vi "Lockin_AIWFM_time.vi"(8 "error in (no error)":errorcluster, 11 "Transport":refnum<class "Transport.lvclass">) -> (0 "error out":errorcluster, 3 "Transport out":refnum<class "Transport.lvclass">)   [LabVIEW 2019, in "Transport.lvclass"]
uses:
  Transport.lvclass
  <userlib>/LevyLab/Instrument Framework/Instrument Types/Cryostat/Instrument.Cryostat.lvclass
  Control Experiment/Control Experiment.lvclass
  Control Experiment/Typedefs/Instrument Classes--cluster.ctl
  <userlib>/LevyLab/Instrument Framework/Instrument Types/VSource/Instrument.VSource.lvclass
  <userlib>/LevyLab/Instrument Framework/Instrument Types/VNA/Instrument.VNA.lvclass
  <userlib>/LevyLab/Instrument Framework/Instrument Types/Strain/Instrument.Strain.lvclass
  <userlib>/LevyLab/Instrument Framework/Instrument Types/CBridge/Instrument.CBridge.lvclass
  <vilib>/Waveform/WDTOps.llb/WDT Append Waveforms DBL.vi
  <vilib>/PRIrvin/XY Utilities/xy_utilities.lvlib
  <vilib>/PRIrvin/XY Utilities/subVIs/Waveform to XY (single).vi
  <vilib>/PRIrvin/XY Utilities/subVIs/Get X and Y (single).vi
  <userlib>/LevyLab/Instrument Framework/Instrument Types/Delay Line/Instrument.DelayLine.lvclass
  <userlib>/LevyLab/Instrument Framework/Instrument Types/Lockin/Instrument.LockinAPI.lvclass
  <userlib>/LevyLab/Instrument Framework/Instrument Types/Amplifier/Instrument.Amplifier.lvclass
panel:
  in  "Stop":bool
  in  "Tab Control":enum32{"Control", "Waveform", "Other"}(tab)
  in  "wait (ms)":u32=1000
  in  "Experiment Description":string="cool down\n\n"
  in  "Experiment Folder":string="cooldown"
  out "AI":cluster{dbl[], dbl[]}[](graph)
  # "*** These controls are only read if this VI is the top level. If is is called from Sweep Control then the folder and comments come from Sweep Control.vi ***"
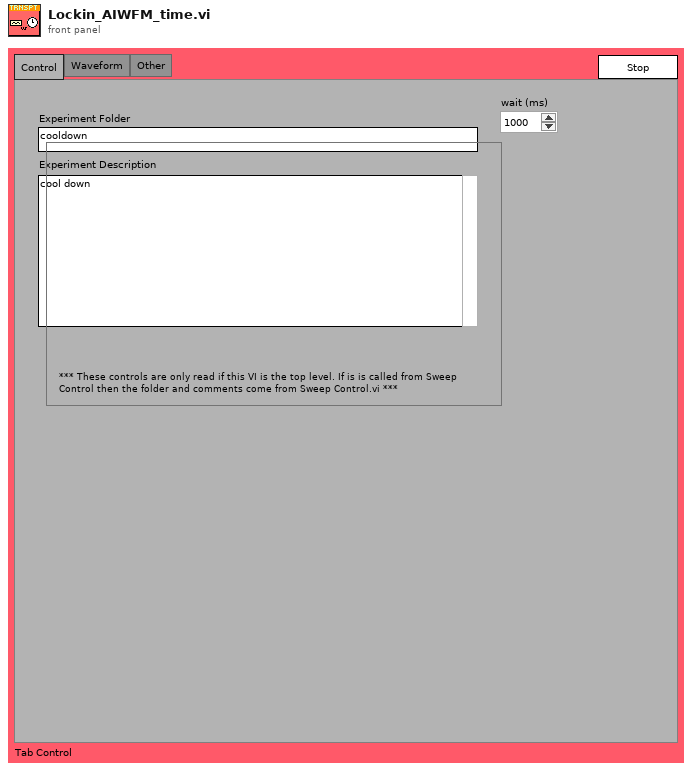
[diagram p1: front panel]
types:
  T1 = enum32{"Invalid", "Standard", "Closed", "Hidden", "Minimized", "Maximized"}
  T2 = enum32{"invalid app kind", "Development System", "Run Time System", "Student Edition", "Embedded LabVIEW", "Evaluation", "Custom"}
  T3 = typedef "Control Experiment.lvclass/Instrument Classes--cluster.ctl" = cluster{"DAQ":refnum<class "Instrument.LockinAPI.lvclass">, "Amplifier":refnum<class "Instrument.Amplifier.lvclass">, "Temperature":refnum<class "Instrument.Cryostat.lvclass">, "Magnet":refnum<class "Instrument.Cryostat.lvclass">, "Rotator":refnum<class "Instrument.Cryostat.lvclass">, "Level":refnum<class "Instrument.Cryostat.lvclass">, "Capacitance":refnum<class "Instrument.CBridge.lvclass">, "Delay Line":refnum<class "Instrument.DelayLine.lvclass">, "Strain Cell":refnum<class "Instrument.Strain.lvclass">, "VNA":refnum<class "Instrument.VNA.lvclass">, "Source":refnum<class "Instrument.VSource.lvclass">}
  T4 = cluster{"Core":cluster{"Current VI Reference":refnum<vi>, "Close Panel on Exit?":bool}, "Transport":refnum<class "Transport.lvclass">, "C.E.":refnum<class "Control Experiment.lvclass">, "Notifier":refnum<notifier>, "Instruments":T3, "path":path, "time":dbl, "temperature":dbl, "magnet field":dbl, "AI XY (new)":cluster{dbl[], dbl[]}[], "AI XY (all)":cluster{dbl[], dbl[]}[], "AI Waveform (s)":waveform(dbl)[], "t0":timestamp, "Execution:State":enum32{"Bad", "Idle", "Run top level", "Running"}}
  T5 = enum32{"Bad", "Idle", "Run top level", "Running"}
  T6 = cluster{"Current VI Reference":refnum<vi>, "Close Panel on Exit?":bool}
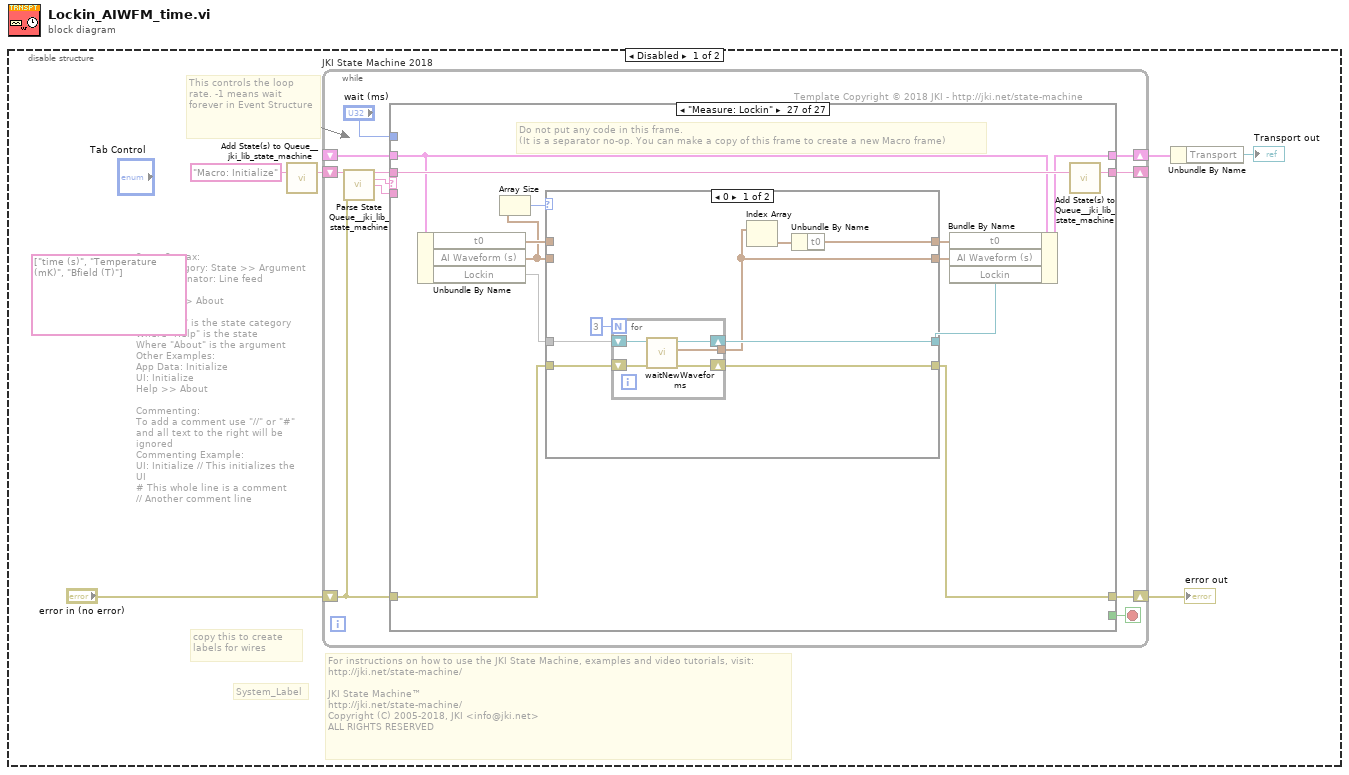
[diagram p0: block diagram]
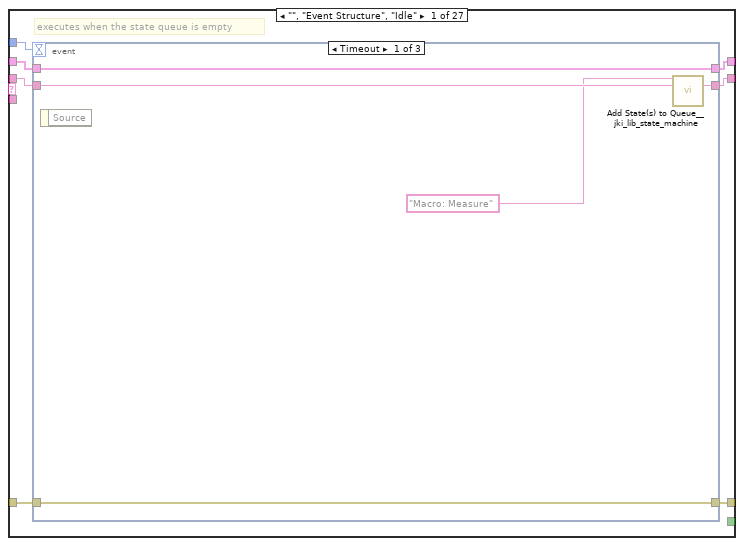
[diagram p2: hidden frame]
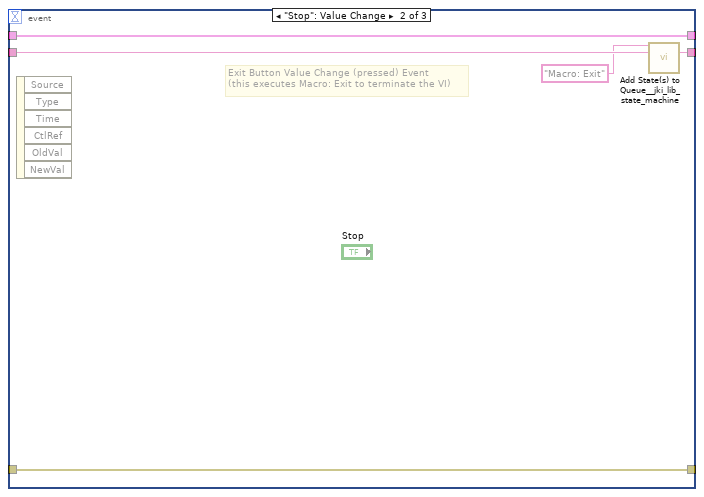
[diagram p3: hidden frame]
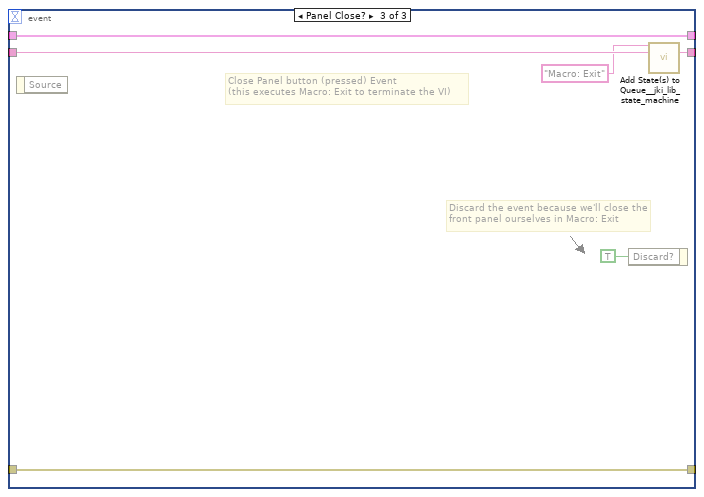
[diagram p4: hidden frame]
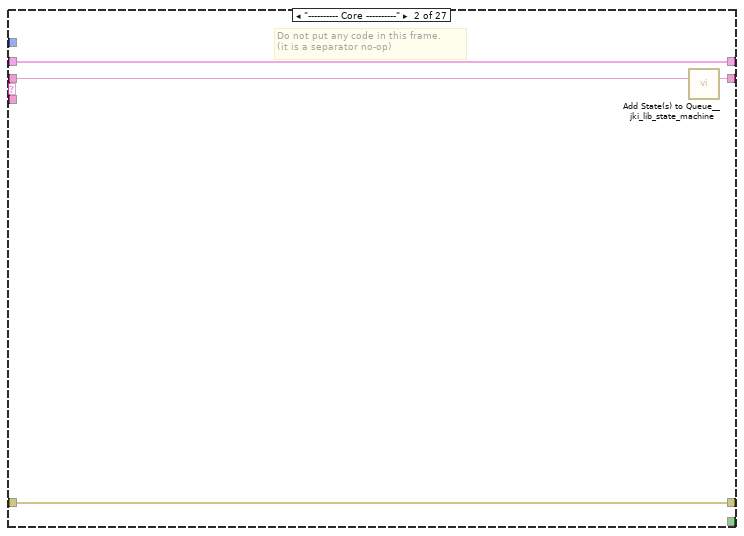
[diagram p5: hidden frame]
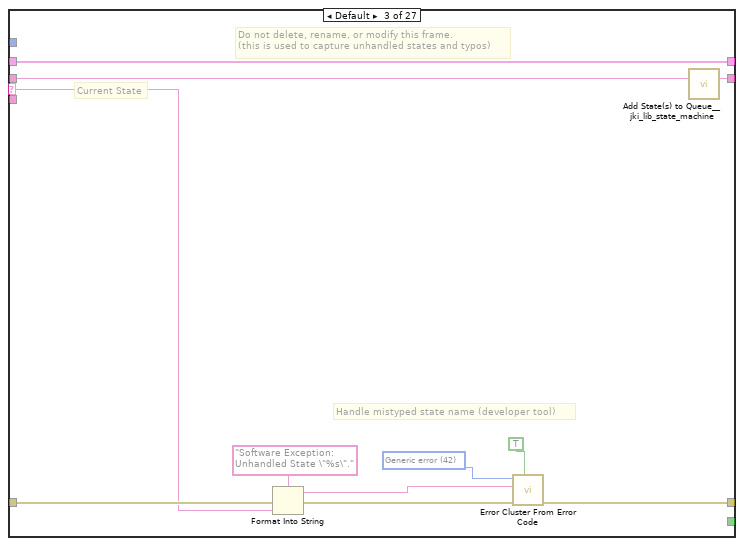
[diagram p6: hidden frame]
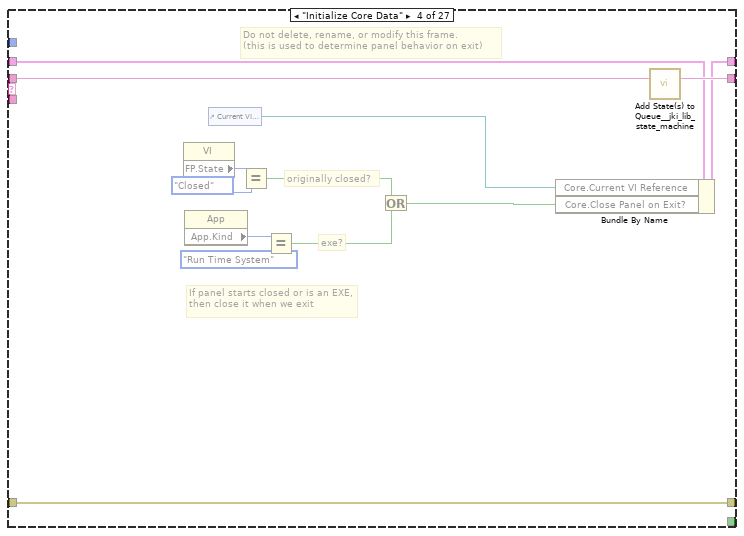
[diagram p7: hidden frame]
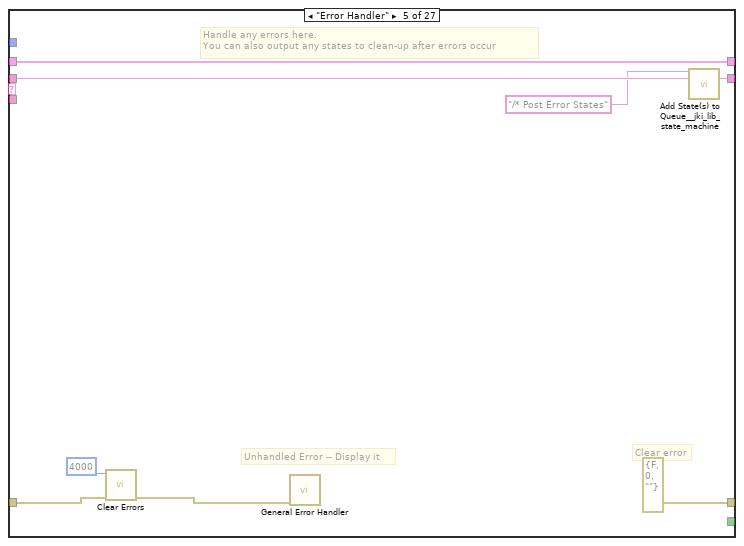
[diagram p8: hidden frame]
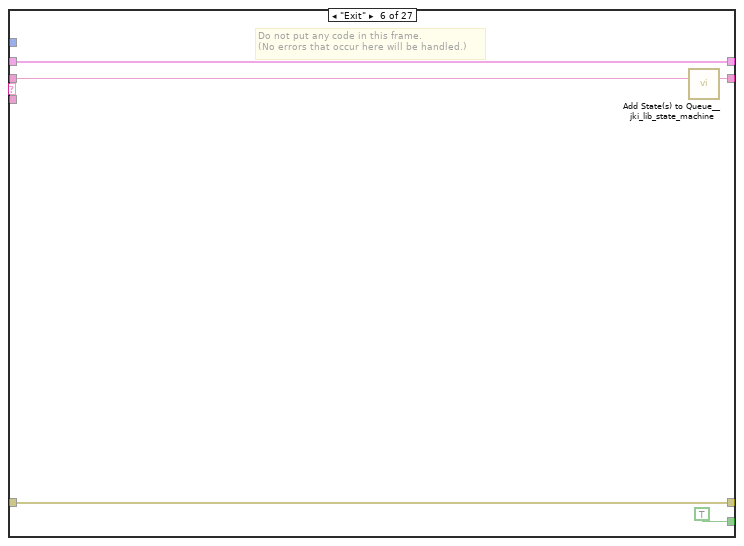
[diagram p9: hidden frame]
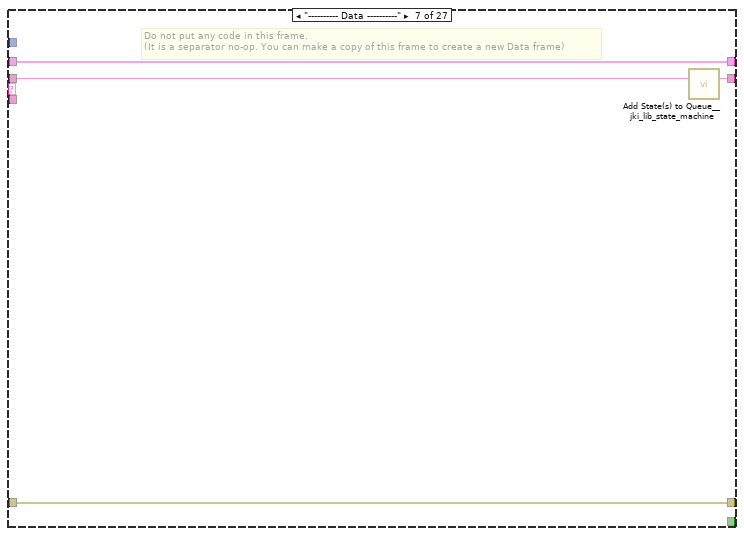
[diagram p10: hidden frame]
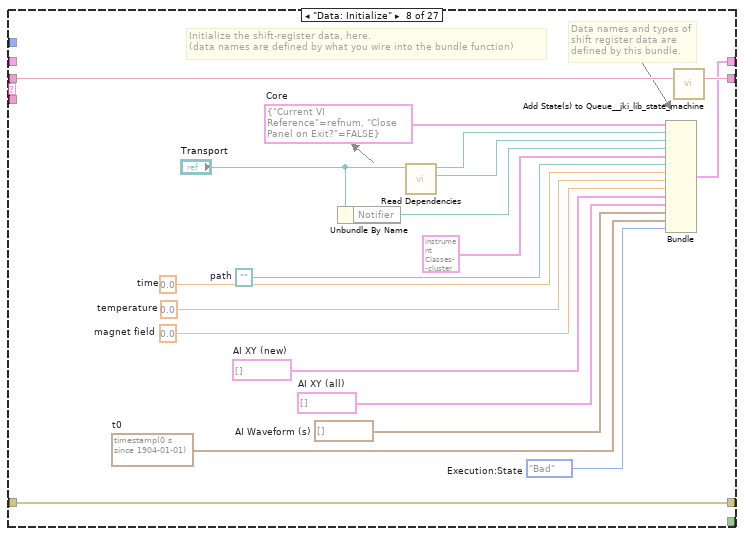
[diagram p11: hidden frame]
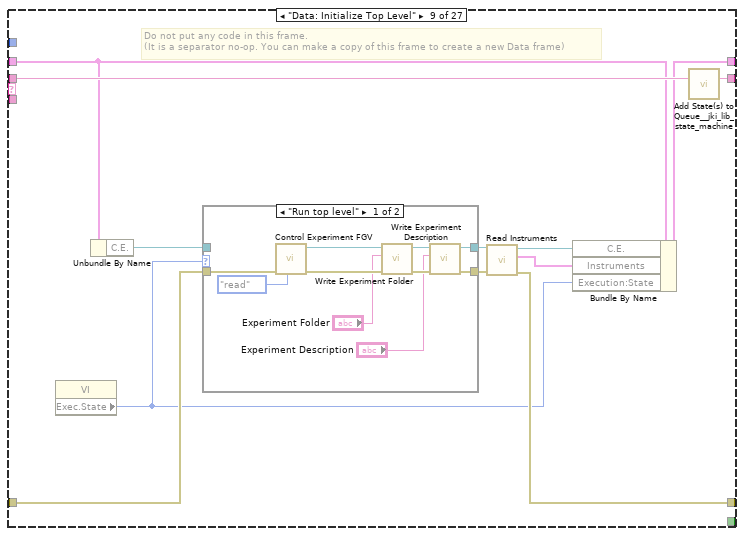
[diagram p12: hidden frame]
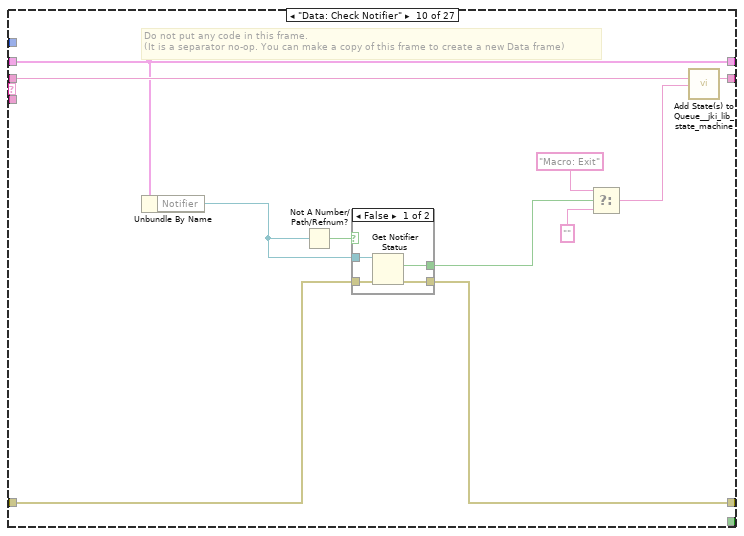
[diagram p14: hidden frame]
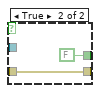
[diagram p15: hidden frame]
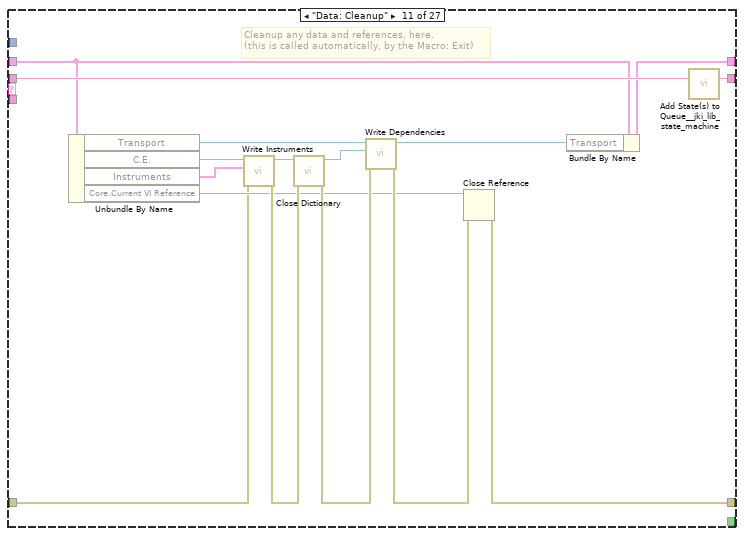
[diagram p16: hidden frame]
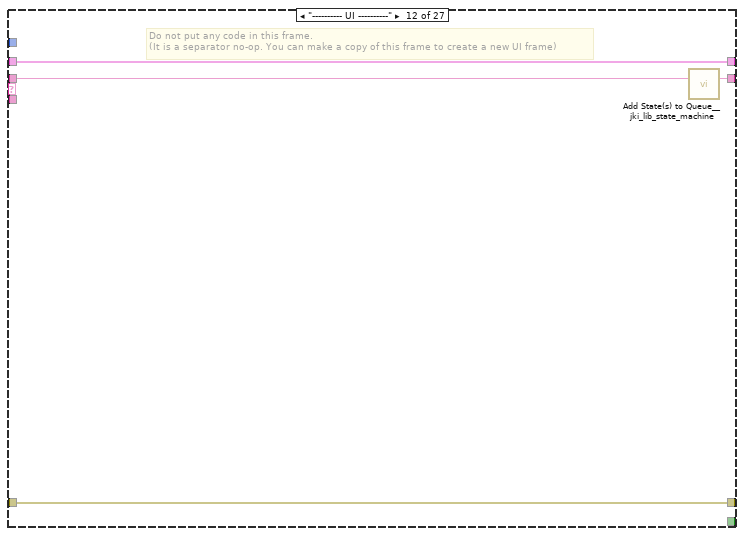
[diagram p17: hidden frame]
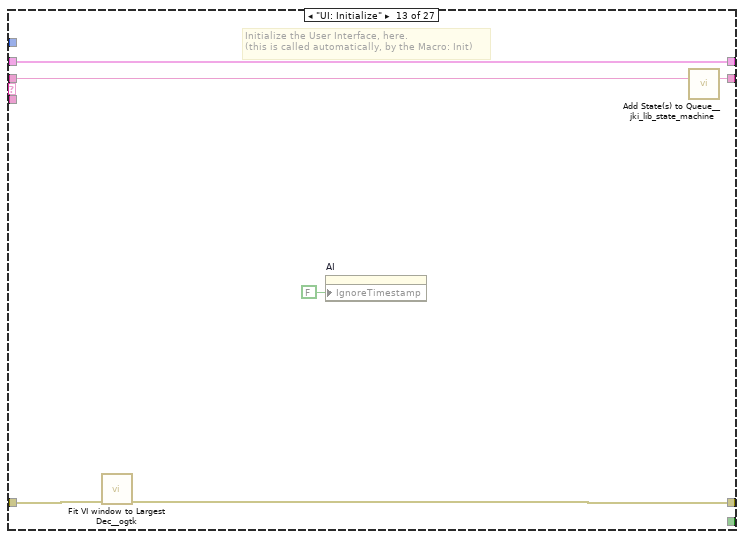
[diagram p18: hidden frame]
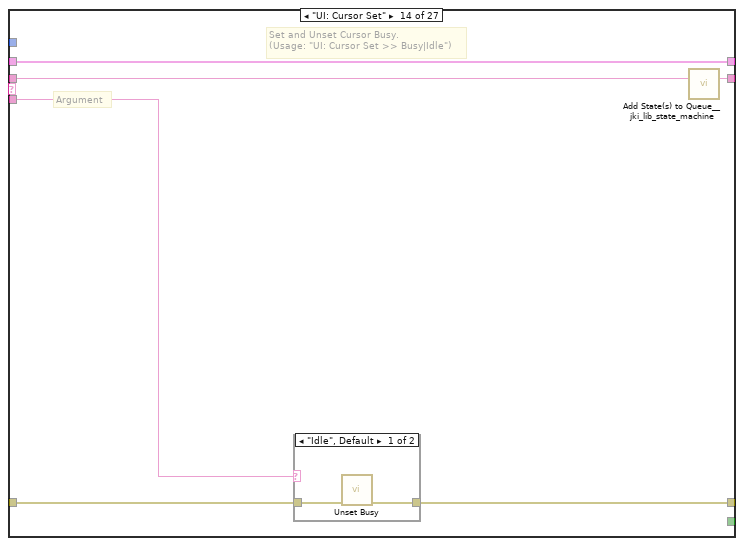
[diagram p19: hidden frame]
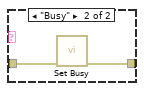
[diagram p20: hidden frame]
diagram:
  n1 = disable-structure shown="Disabled" {
    frame Disabled {
      (unwired) string[] ["time (s)", "Temperature (mK)", "Bfield (T)"] ("wavenames (.Vx, etc)")
      # "For instructions on how to use the JKI State Machine, examples and video tutorials, visit:\nhttp://jki.net/state-machine/\n\nJKI State Machine™\nhttp://jki.net/state-machine/\nCopyright (C) 2005-2018, JKI <info@jki.net>\nALL RIGHTS RESERVED"
      # "State Syntax:\nStateCategory: State >> Argument\nLine Terminator: Line feed\nExample:\nUI: Help >> About\n\nWhere \"UI\" is the state category\nWhere \"Help\" is the state\nWhere \"About\" is the argument\nOther Examples:\nApp Data: Initialize\nUI: Initialize\nHelp >> About\n\nCommenting:\nTo add a comment use \"//\" or \"#\" and all text to the right will be ignored\nCommenting Example:\nUI: Initialize // This initializes the UI\n# This whole line is a comment\n// Another comment line"
      # "copy this to create labels for wires"
      # "This controls the loop rate. -1 means wait forever in Event Structure"
      # "System_Label"
      n2 = call <vilib>:"Add State(s) to Queue__jki_lib_state_machine.vi"("State(s) in (\"\")"="Macro: Initialize") -> ("States Out"=w6:string)  [unwired: 14 in]
      n3 = while "JKI State Machine 2018" {
        shift-right: [w10] -> w2
        shift-left: _ -> [w9]
        shift-right: [w13] -> w3
        shift-left: "error in (no error)" -> [w8]
        shift-right: [w12] -> _
        shift-left: w6 -> [w14]
        stop <- w11 stop-if-true
        # "Template Copyright © 2018 JKI - http://jki.net/state-machine"
        n4 = call <vilib>:"Parse State Queue__jki_lib_state_machine.vi"("State Queue"=w14, "Error In (no error)"=w8) -> ("Remaining States"=w16:string, "Current State"=w17:string, "Arguments"=w15:string)  [unwired: 11 in]
        n5 = case shown="\"Measure: Lockin\"" w17 {
          selector: w17 -> [_ _ w45 _ _ _ _ _ _ _ _ _ _ _ _ _ _ _ _ _ _ _ _ _ _ _ _]
          tunnel: w16 -> [w24 w44 w49 w68 w76 w81 w85 w104 w116 w139 w161 w165 w171 w177 w188 w258 w262 w267 w275 w285 w289 w303 w327 w338 w351 w364 w377]
          tunnel: w15 -> [_ _ _ _ _ _ _ _ _ _ _ _ _ w172 w182 _ _ _ _ _ _ _ _ _ _ _ _]
          tunnel: w9 -> [w22 w41 w47 w61 w73 w79 w82 _ w112 w136 w146 w162 w169 w175 w184 w256 w259 w264 w272 w282 w286 w292 w324 w334 w347 w362 w374]
          tunnel: [w21 w42 w51 w65 errorcluster {"status"=FALSE, "code"=0, "source"=""} ("error out") w78 w83 w101 w106 w135 w148 w163 w167 w173 w185 w255 w260 w265 w273 w283 w287 w301 w325 w328 w340 w357 w368] -> w13
          tunnel: w8 -> [w20 w42 w50 w65 w70 w78 w83 w101 w111 w134 w149 w163 w168 w174 w186 w255 w260 w265 w273 w283 w287 w296 w325 w331 w348 w356 w369]
          tunnel: [w23 w43 w48 w67 w75 w80 w84 w103 w115 w138 w160 w164 w170 w176 w187 w257 w261 w266 w274 w284 w288 w302 w326 w337 w350 w363 w376] -> w12
          tunnel: [_ _ _ _ _ TRUE _ _ _ _ _ _ _ _ _ _ _ _ _ _ _ _ _ _ _ _ _] -> w11
          tunnel: [w19 w41 w47 w66 w73 w79 w82 w102 w113 w136 w147 w162 w169 w175 w184 w256 w259 w264 w272 w282 w286 w291 w324 w335 w346 w361 w375] -> w10
          tunnel: "wait (ms)" -> [w18 _ _ _ _ _ _ _ _ _ _ _ _ _ _ _ _ _ _ _ _ _ _ _ _ _ _]
          frame "", "Event Structure", "Idle" {
            # "executes when the state queue is empty"
            n6 = event shown="[0] Timeout" {
              selector: _ -> [_ _ _]
              dyn-events: _ -> [_ _ _]
              timeout: w18 -> [_ _ _]
              tunnel: w24 -> [w29 w34 w40]
              tunnel: [w28 w33 w39] -> w23
              tunnel: w22 -> [w26 w31 w37]
              tunnel: [w27 w32 w38] -> w21
              tunnel: w20 -> [w27 w32 w38]
              tunnel: [w26 w31 w37] -> w19
              event Timeout {
                n7 = event-data() -> ()  [unwired: 1 in, 1 out]
                n8 = call <vilib>:"Add State(s) to Queue__jki_lib_state_machine.vi"("State(s) in Front (\"\")"="Macro: Measure" ("State(s) in Front (\"\")"), "State(s) in (\"\")"=w29) -> ("States Out"=w28:string)  [unwired: 13 in]
              }
              event "Stop": Value Change {
                # "Exit Button Value Change (pressed) Event\n(this executes Macro: Exit to terminate the VI)"
                n9 = event-data() -> ()  [unwired: 1 in, 6 out]
                n10 = call <vilib>:"Add State(s) to Queue__jki_lib_state_machine.vi"("State(s) in Front (\"\")"="Macro: Exit", "State(s) in (\"\")"=w34) -> ("States Out"=w33:string)  [unwired: 13 in]
              }
              event Panel Close? {
                # "Discard the event because we'll close the front panel ourselves in Macro: Exit"
                # "Close Panel button (pressed) Event\n(this executes Macro: Exit to terminate the VI)"
                n11 = event-data() -> ()  [unwired: 1 in, 1 out]
                n12 = event-data("Discard?"=TRUE) -> ()  [unwired: 1 in, 1 out]
                n13 = call <vilib>:"Add State(s) to Queue__jki_lib_state_machine.vi"("State(s) in Front (\"\")"="Macro: Exit", "State(s) in (\"\")"=w40) -> ("States Out"=w39:string)  [unwired: 13 in]
              }
            }
          }
          frame "---------- Core ----------" {
            # "Do not put any code in this frame.\n(it is a separator no-op)"
            n14 = call <vilib>:"Add State(s) to Queue__jki_lib_state_machine.vi"("State(s) in (\"\")"=w44) -> ("States Out"=w43:string)  [unwired: 14 in]
          }
          frame Default {
            w54 = 42 items=["No error", "Argument error", "Memory is full", "Out of zone", "End of file", "File already open", "Generic file I/O error", "File not found", "File permission error", "Disk is full", "Duplicate path", "Too many files open", "System feature not enabled", "Resource file not found", "Cannot add resource", "Resource not found", "Image not found", "Image memory error", "Pen does not exist", "Config type invalid", "Config token not found", "Config parse error", "Config memory error", "Bad external code format", "Bad external code offset", "External code not present", "Null window", "Destroy window error", "Null menu", "Print aborted", "Bad print record", "Print driver error", "Windows error during printing", "Memory error during printing", "Print dialog error", "Generic print error", "Invalid device refnum", "Device not found", "Device parameter error", "Device unit error", "Cannot open device", "Device call aborted", "Generic error", "Cancelled by user", "Object ID too low", "Object ID too high", "Object not in heap", "Unknown heap", "Unknown object (invalid DefProc)", "Unknown object (DefProc not in table)", "Message out of range", "Invalid (null) method", "Unknown message", "Manager call not supported", "Bad address", "Network operation in progress", "Network operation timed out", "Connection is busy", "Network attribute not supported", "Network error", "Address in use", "System out of memory", "Connection aborted", "Connection refused", "Not connected", "Already connected", "Connection closed", "Initialization error (interapplication manager)", "Bad occurrence", "Wait on unbound occurrence handler", "Occurrence queue overflow", "Datalog type conflict", "Unused", "Unrecognized type (interapplication manager)", "Memory corrupt", "Failed to make temporary DLL", "Old CIN version", "Drag socket not found", "Failed to load drop-object", "Failed to register OLE object", "Failed to release OLE object", "Format specifier type mismatch", "Unknown format specifier", "Too few format specifiers", "Too many format specifiers", "Scan failed", "Newer CIN version", "Error converting to variant", "Runtime menu error", "Password tampered", "Variant attribute not found", "Incompatible variant data type", "Event data is not available", "Event Store is not present", "Occurrence is not found", "Event Queue is not created", "Event info is not available", "Refnum passed is NULL", "Error retrieving Class GUID", "Error retrieving CoClass GUID", "Error retrieving TypeLib GUID.", "Bad built application magic bytes.", "Specific driver is different from the specific driver associated with the Logical Name.", "There is no session opened to the class driver.", "Max Error", "MAX - Error with config objects", "MAX - Error loading configuration", "MAX - Group not supported"]
            # "Current State"
            # "Do not delete, rename, or modify this frame.\n(this is used to capture unhandled states and typos)"
            # "Handle mistyped state name (developer tool)"
            n15 = Format Into String(format string="Software Exception: Unhandled State \"%s\"." ("message"), error in=w50, w45) -> (resulting string=w53:string, error out=w52:errorcluster)  [unwired: 1 in]
            n16 = call <vilib>:"Error Cluster From Error Code.vi"("show call chain? (False)"=TRUE, "error in (no error)"=w52, "error message (\"\")"=w53, "error code (0)"=w54) -> ("error out"=w51:errorcluster)  [unwired: 5 in]
            n17 = call <vilib>:"Add State(s) to Queue__jki_lib_state_machine.vi"("State(s) in (\"\")"=w49) -> ("States Out"=w48:string)  [unwired: 14 in]
          }
          frame "Initialize Core Data" {
            # "Do not delete, rename, or modify this frame.\n(this is used to determine panel behavior on exit)"
            # "originally closed?"
            # "exe?"
            # "If panel starts closed or is an EXE, then close it when we exit"
            n18 = property class="VI"() -> ("FP.State"=w58:T1)  [unwired: 2 in, 2 out]
            n19 = property class="App"() -> ("App.Kind"=w64:T2)  [unwired: 2 in, 2 out]
            n20 = control-ref of="Current VI Reference"() -> (w59:refnum<vi>)
            n21 = Equal?(x=w58, y=T1."Closed" ("Front Panel Window:State")) -> (x = y?=w56:bool)
            n22 = Equal?(x=w64, y=T2."Run Time System" ("Application:Kind")) -> (x = y?=w62:bool)
            n23 = Or(x=w56, y=w62) -> (x .or. y?=w60:bool)
            n24 = Bundle By Name(cluster=w61, "Core.Current VI Reference"=w59, "Core.Close Panel on Exit?"=w60) -> (w66:T4)
            n25 = call <vilib>:"Add State(s) to Queue__jki_lib_state_machine.vi"("State(s) in (\"\")"=w68) -> ("States Out"=w67:string)  [unwired: 14 in]
          }
          frame "Error Handler" {
            # "Unhandled Error -- Display it"
            # "Handle any errors here.\nYou can also output any states to clean-up after errors occur"
            # "Clear error"
            n26 = call <vilib>:"Clear Errors.vi"("error in (no error)"=w70, "specific error code to clear (0: all)"=4000) -> ("error out"=w69:errorcluster)  [unwired: 4 in, 1 out]
            n27 = call <vilib>:"General Error Handler.vi"("error in (no error)"=w69) -> ()  [unwired: 10 in, 5 out]
            n28 = call <vilib>:"Add State(s) to Queue__jki_lib_state_machine.vi"("State(s) in Front (\"\")"="/* Post Error States", "State(s) in (\"\")"=w76) -> ("States Out"=w75:string)  [unwired: 13 in]
          }
          frame "Exit" {
            # "Do not put any code in this frame.\n(No errors that occur here will be handled.)"
            n29 = call <vilib>:"Add State(s) to Queue__jki_lib_state_machine.vi"("State(s) in (\"\")"=w81) -> ("States Out"=w80:string)  [unwired: 14 in]
          }
          frame "---------- Data ----------" {
            # "Do not put any code in this frame.\n(It is a separator no-op. You can make a copy of this frame to create a new Data frame)"
            n30 = call <vilib>:"Add State(s) to Queue__jki_lib_state_machine.vi"("State(s) in (\"\")"=w85) -> ("States Out"=w84:string)  [unwired: 14 in]
          }
          frame "Data: Initialize" {
            w89 = T5."Bad"  # Execution:State
            w90 = timestamp(0 s since 1904-01-01)  # t0
            w91 = waveform(dbl)[] []  # AI Waveform (s)
            w96 = cluster{dbl[], dbl[]}[] []  # AI XY (new)
            w97 = cluster{dbl[], dbl[]}[] []  # AI XY (all)
            w94 = 0.0  # magnet field
            w93 = 0.0  # temperature
            w92 = 0.0  # time
            w99 = path ""  # path
            w100 = T6 {"Current VI Reference"=refnum, "Close Panel on Exit?"=FALSE}  # Core
            # "Data names and types of shift register data are defined by this bundle."
            # "Initialize the shift-register data, here.\n(data names are defined by what you wire into the bundle function)"
            n31 = Unbundle By Name("Transport") -> ("Notifier"=w98:refnum<notifier>)
            n32 = call "Read Dependencies.vi"("Transport"="Transport") -> ("C.E."=w86:refnum<class "Control Experiment.lvclass">, "Transport"=w87:refnum<class "Transport.lvclass">)  [unwired: 8 in, 1 out]
            n33 = Bundle("Core"=w100, "Transport"=w87, "C.E."=w86, "Notifier"=w98, "Instruments"=T3 {"DAQ"=refnum, "Amplifier"=refnum, "Temperature"=refnum, "Magnet"=refnum, "Rotator"=refnum, "Level"=refnum, "Capacitance"=refnum, "Delay Line"=refnum, "Strain Cell"=refnum, "VNA"=refnum, "Source"=refnum}, "path"=w99, "time"=w92, "temperature"=w93, "magnet field"=w94, "AI XY (new)"=w96, "AI XY (all)"=w97, "AI Waveform (s)"=w91, "t0"=w90, "Execution:State"=w89) -> (w102:T4)  [unwired: 1 in]
            n34 = call <vilib>:"Add State(s) to Queue__jki_lib_state_machine.vi"("State(s) in (\"\")"=w104) -> ("States Out"=w103:string)  [unwired: 14 in]
          }
          frame "Data: Initialize Top Level" {
            # "Do not put any code in this frame.\n(It is a separator no-op. You can make a copy of this frame to create a new Data frame)"
            n35 = property class="VI"() -> ("Exec.State"=w105:T5)  [unwired: 2 in, 2 out]
            n36 = Unbundle By Name(w112) -> ("C.E."=w114:refnum<class "Control Experiment.lvclass">)
            n37 = case shown="\"Run top level\"" w105 {
              tunnel: w111 -> [w126 w127]
              tunnel: [w121 w127] -> w110
              tunnel: [w120 w128] -> w109
              tunnel: w114 -> [_ w128]
              frame "Run top level" {
                n38 = call "Control Experiment FGV.vi"("Function"=enum16{"read", "write"}."read", "error in (no error)"=w126) -> ("error out"=w124:errorcluster, "Control Experiment.lvclass out"=w125:refnum<class "Control Experiment.lvclass">)  [unwired: 8 in]
                n39 = call "Write Experiment Folder.vi"("error in (no error)"=w124, "Experiment Folder"="Experiment Folder", "Control Experiment in"=w125) -> ("error out"=w122:errorcluster, "Control Experiment out"=w123:refnum<class "Control Experiment.lvclass">)  [unwired: 7 in]
                n40 = call "Write Experiment Description.vi"("error in (no error)"=w122, "Experiment Description"="Experiment Description", "Control Experiment in"=w123) -> ("error out"=w121:errorcluster, "Control Experiment out"=w120:refnum<class "Control Experiment.lvclass">)  [unwired: 7 in]
              }
              frame "Running", Default {
              }
            }
            n41 = call "Read Instruments.vi"("error in (no error)"=w110, "Control Experiment in"=w109) -> ("error out"=w106:errorcluster, "Instruments"=w107:T3, "Control Experiment out"=w108:refnum<class "Control Experiment.lvclass">)  [unwired: 7 in]
            n42 = Bundle By Name(cluster=w112, "C.E."=w108, "Instruments"=w107, "Execution:State"=w105) -> (w113:T4)
            n43 = call <vilib>:"Add State(s) to Queue__jki_lib_state_machine.vi"("State(s) in (\"\")"=w116) -> ("States Out"=w115:string)  [unwired: 14 in]
          }
          frame "Data: Check Notifier" {
            # "Do not put any code in this frame.\n(It is a separator no-op. You can make a copy of this frame to create a new Data frame)"
            n44 = Unbundle By Name(w136) -> ("Notifier"=w129:refnum<notifier>)
            n45 = Not A Number/Path/Refnum?(number/path/refnum=w129) -> (NaN/Path/Refnum?=w137:bool)
            n46 = case shown="False" w137 {
              tunnel: [w143 FALSE] -> w133
              tunnel: [w142 w144] -> w135
              tunnel: w129 -> [w141 _]
              tunnel: w134 -> [w140 w144]
              frame False {
                n47 = Get Notifier Status(notifier=w141, error in (no error)=w140) -> (current notification=w143:bool, error out=w142:errorcluster)  [unwired: 3 out]
              }
              frame True {
              }
            }
            n48 = Select(t="Macro: Exit", s=w133, f="") -> (s? t:f=w130:string)
            n49 = call <vilib>:"Add State(s) to Queue__jki_lib_state_machine.vi"("State(s) in (\"\")"=w139, "State(s) at Back (\"\")"=w130) -> ("States Out"=w138:string)  [unwired: 13 in]
          }
          frame "Data: Cleanup" {
            # "Cleanup any data and references, here.\n(this is called automatically, by the Macro: Exit)"
            n50 = Unbundle By Name(w146) -> ("Transport"=w158:refnum<class "Transport.lvclass">, "C.E."=w156:refnum<class "Control Experiment.lvclass">, "Instruments"=w154:T3, "Core.Current VI Reference"=w150:refnum<vi>)
            n51 = call "Write Instruments.vi"("error in (no error)"=w149, "Instruments"=w154, "Control Experiment in"=w156) -> ("error out"=w153:errorcluster, "Control Experiment out"=w155:refnum<class "Control Experiment.lvclass">)  [unwired: 7 in]
            n52 = call "Close Dictionary.vi"("error in (no error)"=w153, "Control Experiment in"=w155) -> ("error out"=w152:errorcluster, "Control Experiment out"=w157:refnum<class "Control Experiment.lvclass">)  [unwired: 8 in]
            n53 = call "Write Dependencies.vi"("error in (no error)"=w152, "Control Experiment"=w157, "Transport in"=w158) -> ("error out"=w151:errorcluster, "Transport out"=w159:refnum<class "Transport.lvclass">)  [unwired: 7 in]
            n54 = Close Reference(reference=w150, error in (no error)=w151) -> (error out=w148:errorcluster)
            n55 = Bundle By Name(cluster=w146, "Transport"=w159) -> (w147:T4)
            n56 = call <vilib>:"Add State(s) to Queue__jki_lib_state_machine.vi"("State(s) in (\"\")"=w161) -> ("States Out"=w160:string)  [unwired: 14 in]
          }
          frame "---------- UI ----------" {
            # "Do not put any code in this frame.\n(It is a separator no-op. You can make a copy of this frame to create a new UI frame)"
            n57 = call <vilib>:"Add State(s) to Queue__jki_lib_state_machine.vi"("State(s) in (\"\")"=w165) -> ("States Out"=w164:string)  [unwired: 14 in]
          }
          frame "UI: Initialize" {
            # "Initialize the User Interface, here.\n(this is called automatically, by the Macro: Init)"
            n58 = call <userlib>:"Fit VI window to Largest Dec__ogtk.vi"("error in (no error)"=w168) -> ("error out"=w167:errorcluster)  [unwired: 5 in, 1 out]
            n59 = property on="AI" class="XYGraph (strict)"("IgnoreTimestamp"=FALSE ("Ignore Timestamp")) -> ()  [unwired: 2 in, 2 out]
            n60 = call <vilib>:"Add State(s) to Queue__jki_lib_state_machine.vi"("State(s) in (\"\")"=w171) -> ("States Out"=w170:string)  [unwired: 14 in]
          }
          frame "UI: Cursor Set" {
            # "Argument"
            # "Set and Unset Cursor Busy.\n(Usage: \"UI: Cursor Set >> Busy|Idle\")"
            n61 = case shown="\"Idle\", Default" w172 {
              tunnel: w174 -> [w179 w181]
              tunnel: [w178 w180] -> w173
              frame "Idle", Default {
                n62 = call <vilib>:"Unset Busy.vi"("error in (no error)"=w179) -> ("error out"=w178:errorcluster)  [unwired: 10 in]
              }
              frame "Busy" {
                n63 = call <vilib>:"Set Busy.vi"("error in (no error)"=w181) -> ("error out"=w180:errorcluster)  [unwired: 9 in, 1 out]
              }
            }
            n64 = call <vilib>:"Add State(s) to Queue__jki_lib_state_machine.vi"("State(s) in (\"\")"=w177) -> ("States Out"=w176:string)  [unwired: 14 in]
          }
          frame "UI: Front Panel State" {
            # "Argument"
            # "Set Front Panel Open or Closed\n(Usage: \"UI: Front Panel State >> Open|Close\")"
            n65 = Unbundle By Name(w184) -> ("Core.Current VI Reference"=w183:refnum<vi>)
            n66 = case shown="\"Minimize\", \"Minimized\"" w182 {
              tunnel: w186 -> [w194 w209 w220 w233 w246]
              tunnel: [w196 w210 w222 w235 w248] -> w185
              tunnel: w183 -> [w195 w207 w221 w234 w247]
              frame "Open", "Standard", Default {
                w189 = T1."Standard" ("State")
                n67 = property class="VI"(reference=w195, error in=w194) -> (reference out=w192:refnum<vi>, error out=w193:errorcluster, "FP.State"=w191:T1)
                n68 = Not Equal?(x=w191, y=w189) -> (x != y?=w190:bool)
                n69 = case shown="True" w190 {
                  tunnel: [w200 w202] -> w196
                  tunnel: w193 -> [w199 w202]
                  tunnel: w192 -> [w198 _]
                  tunnel: w189 -> [w197 _]
                  frame True {
                    n70 = invoke class="VI" method="FP.Open"(reference=w198, error in=w199, "Activate"=TRUE, "State"=w197) -> (error out=w200:errorcluster)  [unwired: 1 in, 4 out]
                  }
                  frame False {
                  }
                }
              }
              frame "Close", "Closed" {
                n71 = property class="VI"(reference=w207, error in=w209) -> (reference out=w206:refnum<vi>, error out=w208:errorcluster, "FP.State"=w204:T1)
                n72 = Not Equal?(x=w204, y=T1."Closed" ("Front Panel Window:State")) -> (x != y?=w203:bool)
                n73 = case shown="True" w203 {
                  tunnel: [w211 w214] -> w210
                  tunnel: w208 -> [w211 w213]
                  tunnel: w206 -> [_ w212]
                  frame False {
                  }
                  frame True {
                    n74 = invoke class="VI" method="FP.Close"(reference=w212, error in=w213) -> (error out=w214:errorcluster)  [unwired: 1 in, 2 out]
                  }
                }
              }
              frame "Hidden", "Hide" {
                w215 = T1."Hidden" ("State")
                n75 = property class="VI"(reference=w221, error in=w220) -> (reference out=w218:refnum<vi>, error out=w219:errorcluster, "FP.State"=w217:T1)
                n76 = Not Equal?(x=w217, y=w215) -> (x != y?=w216:bool)
                n77 = case shown="True" w216 {
                  tunnel: [w226 w227] -> w222
                  tunnel: w219 -> [w225 w227]
                  tunnel: w218 -> [w224 _]
                  tunnel: w215 -> [w223 _]
                  frame True {
                    n78 = invoke class="VI" method="FP.Open"(reference=w224, error in=w225, "State"=w223) -> (error out=w226:errorcluster)  [unwired: 2 in, 4 out]
                  }
                  frame False {
                  }
                }
              }
              frame "Minimize", "Minimized" {
                w228 = T1."Minimized" ("State")
                n79 = property class="VI"(reference=w234, error in=w233) -> (reference out=w231:refnum<vi>, error out=w232:errorcluster, "FP.State"=w230:T1)
                n80 = Not Equal?(x=w230, y=w228) -> (x != y?=w229:bool)
                n81 = case shown="True" w229 {
                  tunnel: [w239 w240] -> w235
                  tunnel: w232 -> [w238 w240]
                  tunnel: w231 -> [w237 _]
                  tunnel: w228 -> [w236 _]
                  frame True {
                    n82 = invoke class="VI" method="FP.Open"(reference=w237, error in=w238, "State"=w236) -> (error out=w239:errorcluster)  [unwired: 2 in, 4 out]
                  }
                  frame False {
                  }
                }
              }
              frame "Maximize", "Maximized" {
                w241 = T1."Maximized" ("State")
                n83 = property class="VI"(reference=w247, error in=w246) -> (reference out=w244:refnum<vi>, error out=w245:errorcluster, "FP.State"=w243:T1)
                n84 = Not Equal?(x=w243, y=w241) -> (x != y?=w242:bool)
                n85 = case shown="True" w242 {
                  tunnel: [w252 w253] -> w248
                  tunnel: w245 -> [w251 w253]
                  tunnel: w244 -> [w250 _]
                  tunnel: w241 -> [w249 _]
                  frame True {
                    n86 = invoke class="VI" method="FP.Open"(reference=w250, error in=w251, "State"=w249) -> (error out=w252:errorcluster)  [unwired: 2 in, 4 out]
                  }
                  frame False {
                  }
                }
              }
            }
            n87 = call <vilib>:"Add State(s) to Queue__jki_lib_state_machine.vi"("State(s) in (\"\")"=w188) -> ("States Out"=w187:string)  [unwired: 14 in]
          }
          frame "UI: Update Graphs" {
            # "Do not put any code in this frame.\n(It is a separator no-op. You can make a copy of this frame to create a new UI frame)"
            n88 = Unbundle By Name(w256) -> ("AI XY (all)"=→"AI":cluster{dbl[], dbl[]}[])
            n89 = call <vilib>:"Add State(s) to Queue__jki_lib_state_machine.vi"("State(s) in (\"\")"=w258) -> ("States Out"=w257:string)  [unwired: 14 in]
          }
          frame "---------- Macro ----------" {
            # "Do not put any code in this frame.\n(It is a separator no-op. You can make a copy of this frame to create a new Macro frame)"
            n90 = call <vilib>:"Add State(s) to Queue__jki_lib_state_machine.vi"("State(s) in (\"\")"=w262) -> ("States Out"=w261:string)  [unwired: 14 in]
          }
          frame "Macro: Initialize" {
            w263 = "Data: Initialize\nInitialize Core Data\nUI: Initialize\nUI: Front Panel State >> Open\nData: Initialize Top Level"  # Data: Initialize Initialize Core Data UI: Initialize UI: Front Panel State >> Open Data: Initialize Top Level
            # "Initialization Macro\n(This is called once, when the VI starts)"
            n91 = call <vilib>:"Add State(s) to Queue__jki_lib_state_machine.vi"("State(s) in Front (\"\")"=w263, "State(s) in (\"\")"=w267) -> ("States Out"=w266:string)  [unwired: 13 in]
          }
          frame "Macro: Measure" {
            # "Initialization Macro\n(This is called once, when the VI starts)"
            n92 = call <vilib>:"Add State(s) to Queue__jki_lib_state_machine.vi"("State(s) in Front (\"\")"="Measure: Time\nMeasure: Temperature\nMeasure: Magnet\nMeasure: Lockin\nUI: Update Graphs", "State(s) in (\"\")"="File: Save", "State(s) at Back (\"\")"="Data: Check Notifier") -> ("States Out"=w270:string)  [unwired: 12 in]
            n93 = call <vilib>:"Add State(s) to Queue__jki_lib_state_machine.vi"("State(s) in Front (\"\")"=w270, "State(s) in (\"\")"=w275) -> ("States Out"=w274:string)  [unwired: 13 in]
          }
          frame "Macro: Exit" {
            # "Exit Macro\n(This is called once, when the VI exits)"
            n94 = Unbundle By Name(w282) -> ("Core.Close Panel on Exit?"=w281:bool)
            n95 = Select(t="UI: Front Panel State >> Close", s=w281, f="") -> (s? t:f=w278:string)
            n96 = call <vilib>:"Add State(s) to Queue__jki_lib_state_machine.vi"("State(s) in (\"\")"=w278, "State(s) at Back (\"\")"="Data: Cleanup\nExit") -> ("States Out"=w276:string)  [unwired: 13 in]
            n97 = call <vilib>:"Add State(s) to Queue__jki_lib_state_machine.vi"("State(s) in Front (\"\")"=w276, "State(s) in (\"\")"=w285) -> ("States Out"=w284:string)  [unwired: 13 in]
          }
          frame "---------- File ----------" {
            # "Template Separator\n(You can make a copy of, or modify, this frame)"
            n98 = call <vilib>:"Add State(s) to Queue__jki_lib_state_machine.vi"("State(s) in (\"\")"=w289) -> ("States Out"=w288:string)  [unwired: 14 in]
          }
          frame "File: Save" {
            # "Your code here.\n(You can make a copy of, or modify, this frame)"
            n99 = Unbundle By Name(w292) -> ("Execution:State"=w294:T5, "C.E."=w298:refnum<class "Control Experiment.lvclass">, "AI Waveform (s)"=w299:waveform(dbl)[])
            n100 = for {
              tunnel: w299 -> [w321] mode=indexing
              tunnel: w296 -> [w320]
              shift-right: [w305] -> w297
              shift-left: w298 -> [w316]
              tunnel: [w304] -> w295
              i -> [w313]
              n101 = call-poly <vilib>:"Waveform to XY.vi"("error in (no error)"=w320, "Waveform in"=w321) -> ("error out"=w322:errorcluster, "XY-data out"=w323:cluster{"X-array":dbl[], "Y-array":dbl[]})  [unwired: 8 in]
              n102 = Increment(x=w313) -> (x+1=w315:i32)
              n103 = call-poly <vilib>:"Get X and Y.vi"("error in (no error)"=w322, "XY-data"=w323) -> ("error out"=w307:errorcluster, "Y-array"=w308:dbl[], "X-array"=w309:dbl[])  [unwired: 6 in, 1 out]
              n104 = Format Into String(format string="Ch%d" ("wavenames"), w315) -> (resulting string=w312:string)  [unwired: 2 in, 1 out]
              n105 = Concatenate Strings(w312, "_x" ("string")) -> (w318:string)
              n106 = call "Write Dictionary Element.vi"("error in (no error)"=w307, "value"=w309, "key"=w318, "Control Experiment in"=w316) -> ("error out"=w306:errorcluster, "Control Experiment out"=w317:refnum<class "Control Experiment.lvclass">)  [unwired: 6 in]
              n107 = Concatenate Strings(w312, "_y" ("string")) -> (w319:string)
              n108 = call "Write Dictionary Element.vi"("error in (no error)"=w306, "value"=w308, "key"=w319, "Control Experiment in"=w317) -> ("error out"=w304:errorcluster, "Control Experiment out"=w305:refnum<class "Control Experiment.lvclass">)  [unwired: 6 in]
            }
            n109 = call "Exec State to Append.vi"("Execution:State"=w294) -> ("append?"=w290:bool)  [unwired: 2 in]
            n110 = call "Save Transport TDMS File.vi"("append?"=w290, "error in (no error)"=w295, "Control Experiment in"=w297) -> ("error out"=w300:errorcluster, "Control Experiment out"=w293:refnum<class "Control Experiment.lvclass">)  [unwired: 7 in]
            n111 = Bundle By Name(cluster=w292, "C.E."=w293) -> (w291:T4)
            n112 = call <vilib>:"Clear Errors.vi"("error in (no error)"=w300) -> ("error out"=w301:errorcluster)  [unwired: 5 in, 1 out]
            n113 = call <vilib>:"Add State(s) to Queue__jki_lib_state_machine.vi"("State(s) in (\"\")"=w303) -> ("States Out"=w302:string)  [unwired: 14 in]
          }
          frame "---------- Measure ----------" {
            # "Do not put any code in this frame.\n(It is a separator no-op. You can make a copy of this frame to create a new Macro frame)"
            n114 = call <vilib>:"Add State(s) to Queue__jki_lib_state_machine.vi"("State(s) in (\"\")"=w327) -> ("States Out"=w326:string)  [unwired: 14 in]
          }
          frame "Measure: Time" {
            # "Do not put any code in this frame.\n(It is a separator no-op. You can make a copy of this frame to create a new Macro frame)"
            n115 = Unbundle By Name(w334) -> ("C.E."=w333:refnum<class "Control Experiment.lvclass">)
            n116 = Get Date/Time In Seconds() -> (seconds since 1Jan1904=w336:timestamp)
            n117 = To Double Precision Float(number=w336) -> (double precision float=w329:dbl)
            n118 = call "Append Dictionary Element.vi"("error in (no error)"=w331, "value"=w329, "key"="Time", "Control Experiment in"=w333) -> ("error out"=w328:errorcluster, "Control Experiment out"=w332:refnum<class "Control Experiment.lvclass">)  [unwired: 6 in]
            n119 = Bundle By Name(cluster=w334, "C.E."=w332) -> (w335:T4)
            n120 = call <vilib>:"Add State(s) to Queue__jki_lib_state_machine.vi"("State(s) in (\"\")"=w338) -> ("States Out"=w337:string)  [unwired: 14 in]
          }
          frame "Measure: Temperature" {
            # "Do not put any code in this frame.\n(It is a separator no-op. You can make a copy of this frame to create a new Macro frame)"
            n121 = Unbundle By Name(w347) -> ("C.E."=w342:refnum<class "Control Experiment.lvclass">, "Instruments.Temperature"=w349:refnum<class "Instrument.Cryostat.lvclass">)
            n122 = call-dynamic "Get Temperature.vi"("error in (no error)"=w348, "Instrument.Cryostat in"=w349) -> ("error out"=w343:errorcluster, "Temperature (K)"=w344:dbl, "Instrument.Cryostat out"=w339:refnum<class "Instrument.Cryostat.lvclass">)  [unwired: 5 in, 2 out]
            n123 = call "Append Dictionary Element.vi"("error in (no error)"=w343, "value"=w344, "key"="Temperature", "Control Experiment in"=w342) -> ("error out"=w340:errorcluster, "Control Experiment out"=w341:refnum<class "Control Experiment.lvclass">)  [unwired: 6 in]
            n124 = Bundle By Name(cluster=w347, "Instruments.Temperature"=w339, "C.E."=w341) -> (w346:T4)
            n125 = call <vilib>:"Add State(s) to Queue__jki_lib_state_machine.vi"("State(s) in (\"\")"=w351) -> ("States Out"=w350:string)  [unwired: 14 in]
          }
          frame "Measure: Magnet" {
            # "Do not put any code in this frame.\n(It is a separator no-op. You can make a copy of this frame to create a new Macro frame)"
            n126 = Unbundle By Name(w362) -> ("C.E."=w359:refnum<class "Control Experiment.lvclass">, "Instruments.Temperature"=w354:refnum<class "Instrument.Cryostat.lvclass">)
            n127 = call-dynamic "Get Magnet.vi"("error in (no error)"=w356, "Instrument.Cryostat in"=w354) -> ("error out"=w355:errorcluster, "B Field (T)"=w353:dbl, "Instrument.Cryostat out"=w352:refnum<class "Instrument.Cryostat.lvclass">)  [unwired: 5 in, 2 out]
            n128 = call "Append Dictionary Element.vi"("error in (no error)"=w355, "value"=w353, "key"="Magnet", "Control Experiment in"=w359) -> ("error out"=w357:errorcluster, "Control Experiment out"=w358:refnum<class "Control Experiment.lvclass">)  [unwired: 6 in]
            n129 = Bundle By Name(cluster=w362, "Instruments.Magnet"=w352, "C.E."=w358) -> (w361:T4)
            n130 = call <vilib>:"Add State(s) to Queue__jki_lib_state_machine.vi"("State(s) in (\"\")"=w364) -> ("States Out"=w363:string)  [unwired: 14 in]
          }
          frame "Measure: Lockin" {
            # "Do not put any code in this frame.\n(It is a separator no-op. You can make a copy of this frame to create a new Macro frame)"
            n131 = Unbundle By Name(w374) -> ("t0"=w371:timestamp, "AI Waveform (s)"=w367:waveform(dbl)[], "Lockin"=w370)
            n132 = Array Size(array=w367) -> (size(s)=w366:i32)
            n133 = case shown="0" w366 {
              tunnel: w367 -> [_ w402]
              tunnel: [w378 w401] -> w373
              tunnel: [w383 w400] -> w368
              tunnel: w369 -> [w384 w399]
              tunnel: [w380 w395] -> w372
              tunnel: w370 -> [w385 w394]
              tunnel: w371 -> [_ w392]
              tunnel: [w379 w391] -> w365
              frame 0 {
                n134 = for {
                  N: 3 -> [_]
                  tunnel: [w387] -> w378
                  shift-right: [w388] -> w383
                  shift-left: w384 -> [w389]
                  shift-right: [w386] -> w379
                  shift-left: w385 -> [w390]
                  n135 = call-dynamic "waitNewWaveforms.vi"("error in (no error)"=w389, "Instrument.LockinAPI in"=w390) -> ("error out"=w388:errorcluster, "Newest AI Waveform"=w387:waveform(dbl)[], "Instrument.LockinAPI out"=w386:refnum<class "Instrument.LockinAPI.lvclass">)  [unwired: 7 in]
                }
                n136 = Index Array(array=w378) -> (element=w382:waveform(dbl))  [unwired: 1 in]
                n137 = Unbundle By Name(w382) -> ("t0"=w380:timestamp)
              }
              frame Default {
                n138 = call-dynamic "getAIwfm.vi"("error in (no error)"=w399, "Instrument.LockinAPI in"=w394) -> ("error out"=w398:errorcluster, "AI Waveform"=w393:waveform(dbl)[], "Instrument.LockinAPI out"=w391:refnum<class "Instrument.LockinAPI.lvclass">)  [unwired: 7 in]
                n139 = Index Array(array=w393) -> (element=w397:waveform(dbl))  [unwired: 1 in]
                n140 = Unbundle By Name(w397) -> ("t0"=w395:timestamp)
                n141 = Equal?(x=w395, y=w392) -> (x = y?=w396:bool)
                n142 = case shown="False" w396 {
                  tunnel: w402 -> [w404 w421]
                  tunnel: [w407 w421] -> w401
                  tunnel: [w406 w422] -> w400
                  tunnel: w398 -> [w405 w422]
                  tunnel: w393 -> [w408 _]
                  frame False {
                    n143 = Array Size(array=w404) -> (size(s)=w403:i32)
                    n144 = case shown="Default" w403 {
                      tunnel: w408 -> [w410 w415]
                      tunnel: [w410 w414] -> w407
                      tunnel: [w409 w413] -> w406
                      tunnel: w405 -> [w409 w412]
                      tunnel: w404 -> [_ w411]
                      frame 0 {
                      }
                      frame Default {
                        n145 = for {
                          tunnel: w411 -> [w416] mode=indexing
                          tunnel: w415 -> [w420] mode=indexing
                          tunnel: [w419] -> w414 mode=indexing
                          tunnel: [w418] -> w413
                          tunnel: w412 -> [w417]
                          n146 = call-poly <vilib>:"Append Waveforms.vi"("error in (no error)"=w417, "waveform B"=w420, "waveform A"=w416) -> ("error out"=w418:errorcluster, "waveform out"=w419:waveform(dbl))  [unwired: 7 in]
                        }
                      }
                    }
                  }
                  frame True {
                  }
                }
              }
            }
            n147 = Bundle By Name(cluster=w374, "t0"=w372, "AI Waveform (s)"=w373, "Lockin"=w365) -> (w375:T4)
            n148 = call <vilib>:"Add State(s) to Queue__jki_lib_state_machine.vi"("State(s) in (\"\")"=w377) -> ("States Out"=w376:string)  [unwired: 14 in]
          }
        }
      }
      "error out" <- w3
      n149 = Unbundle By Name(w2) -> ("Transport"=→"Transport out":refnum<class "Transport.lvclass">)
    }
    frame Enabled {
    }
  }
